vi "NAV_DRIVE_SIMPLE.vi"(7 "arguments":string[](array[string]), 8 "dt":i32, 9 "Reinit":bool, 10 "bus_inputs":T1, 11 "bus_state":T2) -> (1 "Done":bool, 2 "bus_inputs out":T1, 3 "bus_state out":T2)   [LabVIEW 2013]
uses:
  drivetrain/dt_shift_state.ctl
  structures/bus_state_drivetrain.ctl
  structures/bus_state_collector.ctl
  structures/bus_state.ctl
  structures/bus_inputs.ctl
  collector/collector_shot_cal.ctl
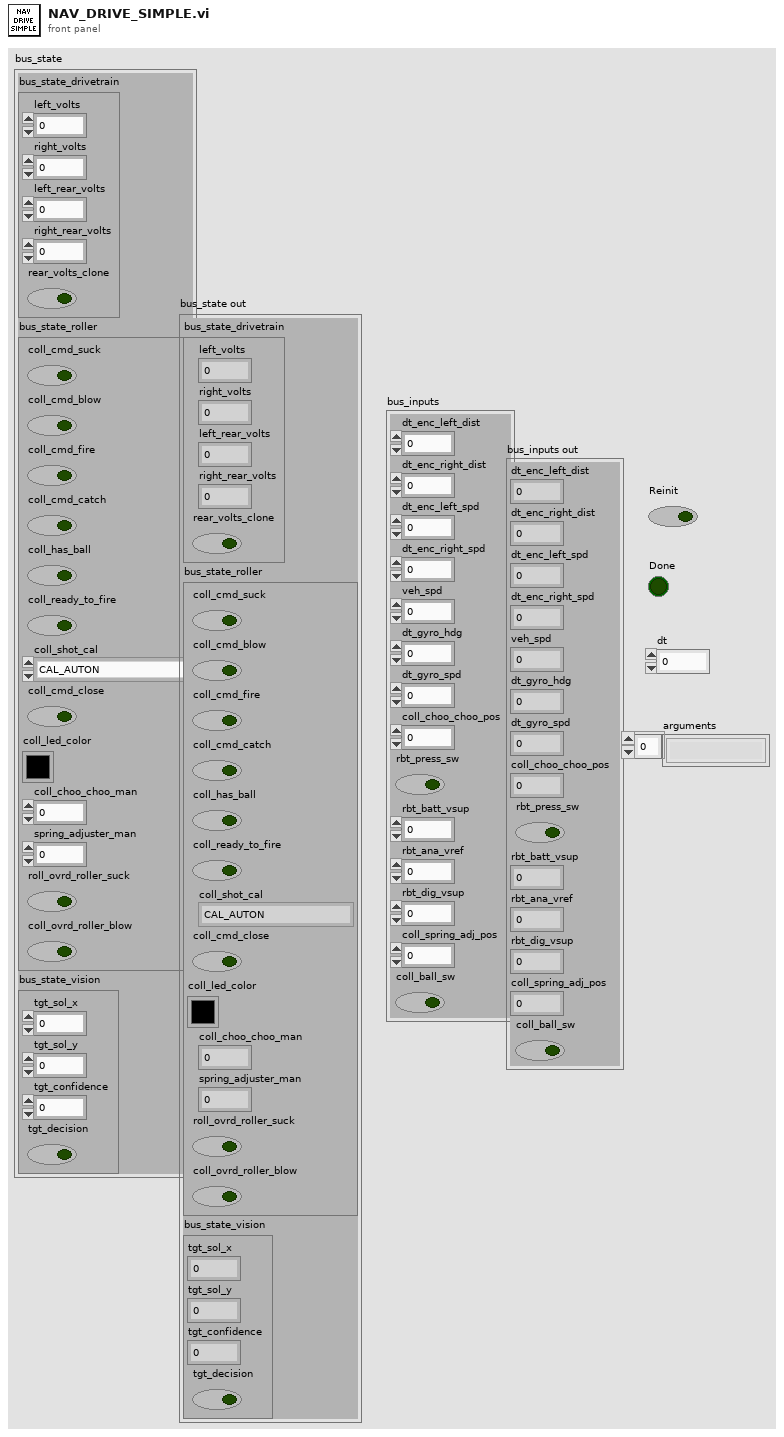
[diagram p1: front panel]
types:
  T1 = typedef "bus_inputs.ctl" = cluster{"dt_enc_left_dist":sgl, "dt_enc_right_dist":sgl, "dt_enc_left_spd":sgl, "dt_enc_right_spd":sgl, "veh_spd":sgl, "dt_gyro_hdg":sgl, "dt_gyro_spd":sgl, "coll_choo_choo_pos":sgl, "rbt_press_sw":bool, "rbt_batt_vsup":sgl, "rbt_ana_vref":dbl, "rbt_dig_vsup":dbl, "coll_spring_adj_pos":sgl, "coll_ball_sw":bool}
  T2 = typedef "bus_state.ctl" = cluster{"bus_state_drivetrain":T3, "bus_state_roller":T4, "bus_state_vision":cluster{"tgt_sol_x":dbl, "tgt_sol_y":dbl, "tgt_confidence":dbl, "tgt_decision":bool}}
  T3 = typedef "bus_state_drivetrain.ctl" = cluster{"left_volts":sgl, "right_volts":sgl, "left_rear_volts":sgl, "right_rear_volts":sgl, "rear_volts_clone":bool}
  T4 = typedef "bus_state_collector.ctl" = cluster{"coll_cmd_suck":bool, "coll_cmd_blow":bool, "coll_cmd_fire":bool, "coll_cmd_catch":bool, "coll_has_ball":bool, "coll_ready_to_fire":bool, "coll_shot_cal":T5, "coll_cmd_close":bool, "coll_led_color":u32, "coll_choo_choo_man":sgl, "spring_adjuster_man":sgl, "roll_ovrd_roller_suck":bool, "coll_ovrd_roller_blow":bool}
  T5 = typedef "collector_shot_cal.ctl" = enum16{"CAL_AUTON", "CAL_CLOSE", "CAL_MID", "CAL_FAR", "NOT_SAFE_TO_ACTUATE"}
  T6 = typedef "dt_shift_state.ctl" = enum16{"low", "high"}
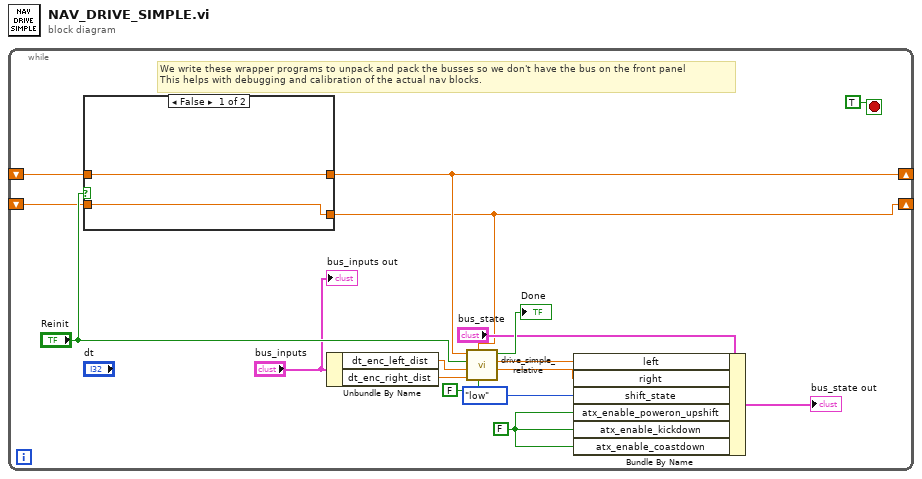
[diagram p0: block diagram]
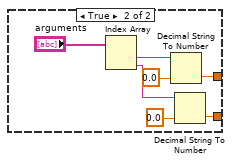
[diagram p2: hidden frame]
diagram:
  n1 = while {
    shift-right: [w15] -> _
    shift-left: _ -> [w16]
    shift-right: [w2] -> _
    shift-left: _ -> [w3]
    stop <- TRUE stop-if-true
    w4 = FALSE ("bus_state_drivetrain.atx_enable_poweron_upshift")
    # "We write these wrapper programs to unpack and pack the busses so we don't have the bus on the front panel\nThis helps with debugging and calibration of the actual nav blocks."
    n2 = case shown="False" "Reinit" {
      tunnel: w16 -> [w19 _]
      tunnel: [w19 w23] -> w15
      tunnel: [w18 w20] -> w2
      tunnel: w3 -> [w18 _]
      frame False {
      }
      frame True {
        n3 = Index Array(array="arguments") -> (element #1=w25:string, element #2=w22:string)  [unwired: 2 in]
        n4 = Decimal String To Number(string=w25, default (0L)=0.0 ("default (0 I32)")) -> (number=w23:dbl)  [unwired: 1 in, 1 out]
        n5 = Decimal String To Number(string=w22, default (0L)=0.0 ("default (0 I32)")) -> (number=w20:dbl)  [unwired: 1 in, 1 out]
      }
    }
    n6 = Unbundle By Name("bus_inputs") -> ("dt_enc_left_dist"=w13:sgl, "dt_enc_right_dist"=w12:sgl)
    n7 = call "drive_simple_relative.vi"("fast"=FALSE, "motor power"=w2, "right distance"=w12, "left distance"=w13, "reinit"="Reinit", "distance target"=w15) -> ("right power"=w7:dbl, "left power"=w8:dbl, "done"=→"Done":bool)  [unwired: 3 in]
    n8 = Bundle By Name(cluster="bus_state", "left"=w8, "right"=w7, "shift_state"=dt_shift_state."low" ("bus_state_drivetrain.shift_state"), "atx_enable_poweron_upshift"=w4, "atx_enable_kickdown"=w4, "atx_enable_coastdown"=w4) -> (→"bus_state out":T2)
    "bus_inputs out" <- "bus_inputs"
  }
